vi "CTR_ControlNodeConfigs.vi"(8 "error in":errorcluster, 10 "StreamCluster_TypeDef in":T1={"DAQ_Configs"=[], "CTR_Config"={"CTR refDes"="", "CTR IP Addr"="", "Restart"=FALSE}, "Network_Configs"={"Buffer"=1, "ManagmentRate_Hz"=1000, "StreamRate_Hz"=10, "ConnectionHysterisis"=0, "LoggingRate_Hz"=10}, "ConfigXML_Checksum"=""}, 11 "DOM document in":refnum<k20>) -> (0 "error out":errorcluster={"status"=TRUE, "code"=-2633, "source"="Property Node (arg 1) in NI_XML.lvlib:Get Node Text Content.vi->CTR_ControlNodeConfigs.vi->CTR_ReadXML_Config.vi->CTRnode.vi"}, 2 "StreamCluster_TypeDef out":T1={"DAQ_Configs"=[], "CTR_Config"={"CTR refDes"="", "CTR IP Addr"="", "Restart"=FALSE}, "Network_Configs"={"Buffer"=1, "ManagmentRate_Hz"=1000, "StreamRate_Hz"=10, "ConnectionHysterisis"=0, "LoggingRate_Hz"=10}, "ConfigXML_Checksum"=""}, 3 "DOM document out":refnum<k20>)   [LabVIEW 2024]
uses:
  Control/StreamCluster_TypeDef.ctl
  Control/streamIO_states.ctl
  <vilib>/xml/Close Reference(Node).vi
  <vilib>/Utility/error.llb/Error Cluster From Error Code.vi
  <vilib>/ErrorRing/Error Ring.xnode
  <vilib>/xml/NI_XML.lvlib
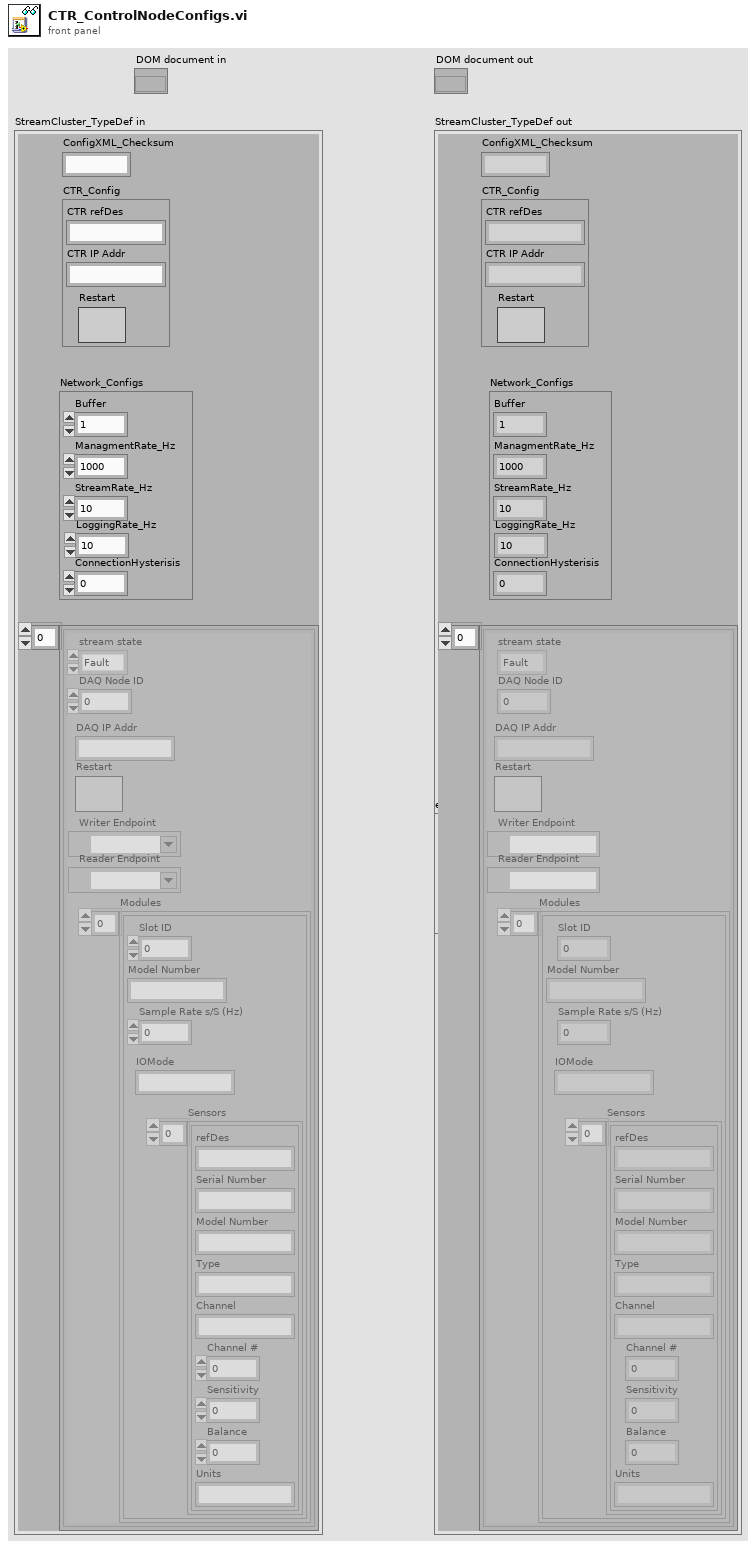
[diagram p1: front panel]
types:
  T1 = typedef "StreamCluster_TypeDef.ctl" = cluster{"DAQ_Configs":cluster{"stream state":T2, "DAQ Node ID":i32, "Writer Endpoint":refnum<k21>, "Reader Endpoint":refnum<k21>, "Modules":cluster{"Slot ID":i32, "Model Number":string, "Sample Rate s/S (Hz)":dbl, "Sensors":cluster{"refDes":string, "Serial Number":string, "Model Number":string, "Type":string, "Channel":string, "Channel #":i32, "Sensitivity":dbl, "Balance":dbl, "Units":string}[], "IOMode":string}[], "DAQ IP Addr":string, "Restart":bool}[], "CTR_Config":cluster{"CTR refDes":string, "CTR IP Addr":string, "Restart":bool}, "Network_Configs":cluster{"Buffer":i32, "ManagmentRate_Hz":i32, "StreamRate_Hz":i32, "ConnectionHysterisis":i32, "LoggingRate_Hz":i32}, "ConfigXML_Checksum":string}
  T2 = typedef "streamIO_states.ctl" = enum16{"Fault", "Initialize", "Stream", "Close"}
  T3 = cluster{"[0]":string, "[1]":string, "[2]":string, "[3]":string, "[4]":string, "[5]":string, "[6]":string, "[7]":string, "[8]":string}
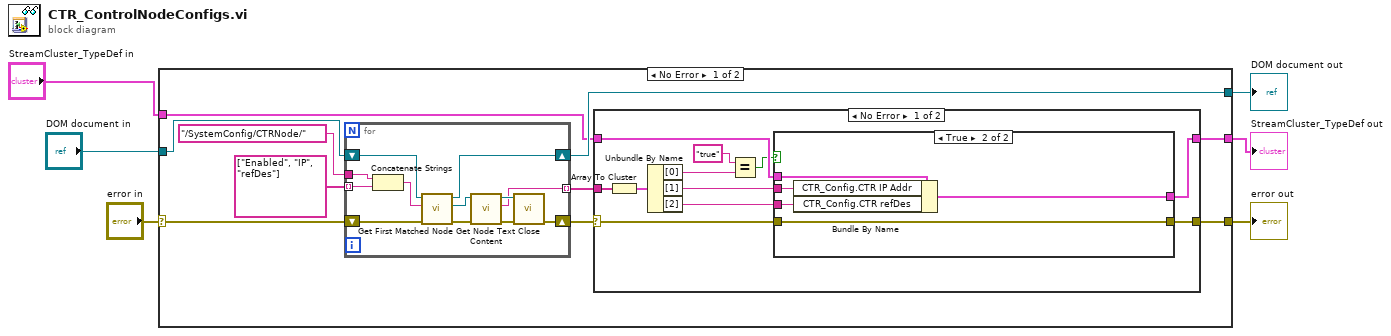
[diagram p0: block diagram]
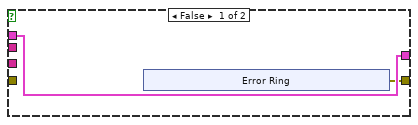
[diagram p2: hidden frame]
diagram:
  n1 = case shown="No Error" "error in" {
    selector: "error in" -> [w16 w56]
    tunnel: [w8 w56] -> w5
    tunnel: "DOM document in" -> [w14 w54]
    tunnel: [w12 w54] -> w3
    tunnel: "StreamCluster_TypeDef in" -> [w10 w55]
    tunnel: [w9 w55] -> w1
    frame No Error {
      n2 = for {
        tunnel: "/SystemConfig/CTRNode/" ("XPath expression") -> [w49]
        tunnel: string[] ["Enabled", "IP", "refDes"] -> [w48] mode=indexing
        shift-right: [w44] -> w12
        shift-left: w14 -> [w50]
        shift-right: [w43] -> w7
        shift-left: w16 -> [w51]
        tunnel: [w42] -> w11 mode=indexing
        n3 = Concatenate Strings(w49, w48) -> (w47:string)
        n4 = call <vilib>:"Get First Matched Node.vi"("error in (no error)"=w51, "XPath expression"=w47, "node in"=w50) -> ("error out"=w52:errorcluster, "node result"=w53:refnum<k20>, "node out"=w44:refnum<k20>)  [unwired: 6 in]
        n5 = call <vilib>:"Get Node Text Content.vi"("error in (no error)"=w52, "node in"=w53) -> ("error out"=w46:errorcluster, "node text"=w42:string, "node out"=w45:refnum<k20>)  [unwired: 7 in]
        n6 = call-poly <vilib>:"Close.vi"("error in (no error)"=w46, "node"=w45) -> ("error out"=w43:errorcluster)  [unwired: 7 out]
      }
      n7 = case shown="No Error" w7 {
        selector: w7 -> [w17 w41]
        tunnel: w11 -> [w27 _]
        tunnel: w10 -> [w25 w40]
        tunnel: [w24 w40] -> w9
        tunnel: [w18 w41] -> w8
        frame No Error {
          n8 = Array To Cluster(array=w27) -> (cluster=w26:T3)
          n9 = Unbundle By Name(w26) -> ("[0]"=w23:string, "[1]"=w20:string, "[2]"=w19:string)
          n10 = Equal?(x="true", y=w23) -> (x = y?=w21:bool)
          n11 = case shown="True" w21 {
            tunnel: w25 -> [w29 w39]
            tunnel: [w29 w38] -> w24
            tunnel: w20 -> [_ w37]
            tunnel: w19 -> [_ w36]
            tunnel: w17 -> [_ w35]
            tunnel: [w28 w35] -> w18
            frame False {
              n12 = xnode "Error Ring"() -> ("error out"=w28:errorcluster)
            }
            frame True {
              n13 = Bundle By Name(cluster=w39, "CTR_Config.CTR IP Addr"=w37, "CTR_Config.CTR refDes"=w36) -> (w38:T1)
            }
          }
        }
        frame Error {
        }
      }
    }
    frame Error {
    }
  }
  "error out" <- w5
  "DOM document out" <- w3
  "StreamCluster_TypeDef out" <- w1
